vi "Find USB-485.vi"() -> (2 "Com Ref":refnum<visa-resource-name>, 3 "485 Found?":bool)   [LabVIEW 2013]
panel:
  out "Array":string[](array[string])
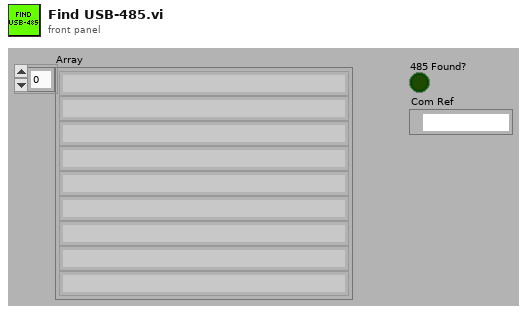
[diagram p1: front panel]
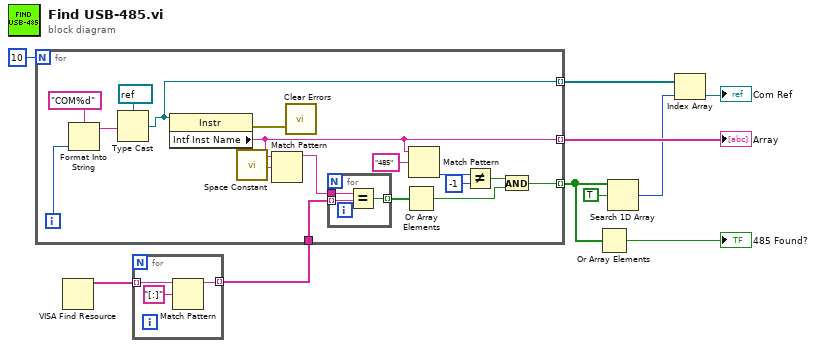
[diagram p0: block diagram]
diagram:
  n1 = VISA Find Resource() -> (3:w2:string[])  [unwired: 3 in, 2 out]
  n2 = for {
    tunnel: w2 -> [w12] mode=indexing
    tunnel: [w11] -> w1 mode=indexing
    n3 = Match Pattern(string=w12, regular expression="[:]") -> (before substring=w11:string)  [unwired: 1 in, 3 out]
  }
  n4 = for {
    N: 10 -> [_]
    tunnel: [w22] -> w10 mode=indexing
    tunnel: [w18] -> w7 mode=indexing
    tunnel: [w17] -> w5 mode=indexing
    tunnel: w1 -> [w16]
    i -> [w29]
    n5 = Format Into String(format string="COM%d", w29) -> (resulting string=w27:string)  [unwired: 2 in, 1 out]
    n6 = Type Cast(type=refnum<visa-resource-name> refnum ("reference"), x=w27) -> (*(type *) &x=w17:refnum<visa-resource-name>)
    n7 = property class="Instr"(reference=w17) -> (error out=w30:errorcluster, "Intf Inst Name"=w22:string)  [unwired: 1 in, 1 out]
    n8 = call <vilib>:"Space Constant.vi"() -> ("String"=w25:string)
    n9 = Match Pattern(string=w22, regular expression=w25) -> (before substring=w24:string)  [unwired: 1 in, 3 out]
    n10 = call <vilib>:"Clear Errors.vi"("error in (no error)"=w30) -> ()  [unwired: 6 in, 1 out]
    n11 = for {
      tunnel: w24 -> [w33]
      tunnel: w16 -> [w32] mode=indexing
      tunnel: [w31] -> w15 mode=indexing
      n12 = Equal?(x=w33, y=w32) -> (x = y?=w31:bool)
    }
    n13 = Or Array Elements(Boolean array=w15) -> (logical OR=w14:bool)
    n14 = Match Pattern(string=w22, regular expression="485") -> (offset past match=w20:i32)  [unwired: 1 in, 3 out]
    n15 = Not Equal?(x=w20, y=-1) -> (x != y?=w19:bool)
    n16 = And(x=w19, y=w14) -> (x .and. y?=w18:bool)
  }
  "Array" <- w10
  n17 = Or Array Elements(Boolean array=w7) -> (logical OR=→"485 Found?":bool)
  n18 = Search 1D Array(1D array=w7, element=TRUE) -> (index of element=w4:i32)  [unwired: 1 in]
  n19 = Index Array(array=w5, index=w4) -> (element=→"Com Ref":refnum<visa-resource-name>)
